vi "GetPicture.vi"() -> ()   [LabVIEW 2009]
panel:
  in  "GetPicture":bool
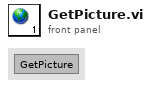
[diagram p1: front panel]
diagram:
